vi "test Inhibit Bus A - Single RT.vi"(8 "error in (no error)":errorcluster, 11 "RT Inhibit Bus A in":refnum<class "RT Inhibit Bus A.lvclass">) -> (0 "error out":errorcluster, 3 "RT Inhibit Bus A out":refnum<class "RT Inhibit Bus A.lvclass">)   [LabVIEW 2016, in "RT Inhibit Bus A.lvclass"]
uses:
  RT Inhibit Bus A.lvclass
  1553 Board/1553 Board.lvclass
  1553 Component/1553 Component.lvclass
  Remote Terminal/Remote Terminal.lvclass
  Remote Terminal/TypeDefs/RT Configuration.ctl
  1553 SubComponent/TypeDefs/Scaling Information.ctl
  1553 SubComponent/1553 SubComponent.lvclass
  1553 SubComponent/TypeDefs/Parameter Table Data.ctl
  Remote Terminal/TypeDefs/Command Type.ctl
  Remote Terminal/TypeDefs/Command Configuration.ctl
  PPLs/FPGA Interface.lvlibp/FPGA Interface/FPGA Interface.lvclass
  D:/SVN/Products/BCI-1553/Software/Development/2016/RealTime/1553 SubComponent/1553 SubComponent.lvclass
  Utilities/FPGA Interface/FPGA Interface.lvclass
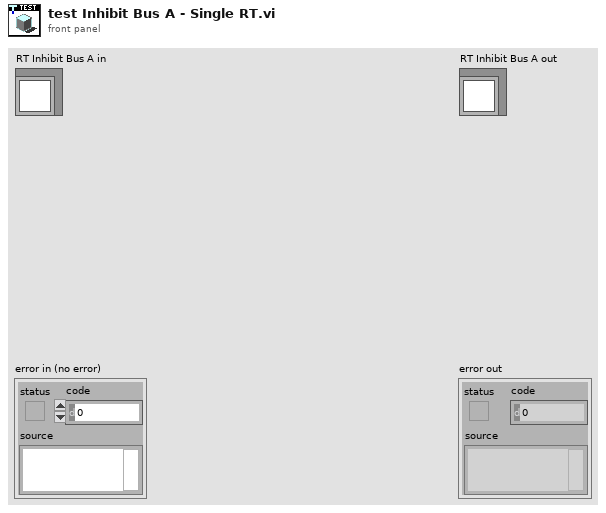
[diagram p1: front panel]
types:
  T1 = typedef "BCI-1553 API.lvlib/Remote Terminal.lvclass/Command Configuration.ctl" = cluster{"Command Type":T2, "Mode Code ID (1-32)":u16, "SubAddress (1-30)":u16, "Word Count (1-32)":u16, "Illegal Command":bool, "Broadcast":bool, "Data":u16[], "Data Fields":T3[]}
  T2 = typedef "BCI-1553 API.lvlib/Remote Terminal.lvclass/Command Type.ctl" = enum16{"Transmit", "Receive", "Mode Code Tx", "Mode Code Rx"}
  T3 = typedef "BCI-1553 API.lvlib/1553 SubComponent.lvclass/Parameter Table Data.ctl" = cluster{"Parameter Name":string, "Base Word":u16, "Address":u16, "Value":u64, "Mask":u16[], "Scaling Info":T4}
  T4 = typedef "BCI-1553 API.lvlib/1553 SubComponent.lvclass/Scaling Information.ctl" = cluster{"Bit Offset":i32, "Bit Count":i32, "LSB Resolution":dbl, "2's Complement":bool, "Big Endian":bool, "Sign Bit":bool}
  T5 = typedef "BCI-1553 API.lvlib/Remote Terminal.lvclass/RT Configuration.ctl" = cluster{"RT-RT TimeOut (us)":u8, "Inhibit Bus A":bool, "Inhibit Bus B":bool, "Broadcast CMD Invalid":bool, "UnDef MCs Invalid":bool, "Notice 2 Data Storage":bool, "SMCP":bool, "Temp RX Buffer":bool, "Alt BIT Enable":bool, "Auto Bus Shutdown":bool, "MC 17 Sync":u8, "MC 16 SR Reset":bool, "MC 8 Reset":bool}
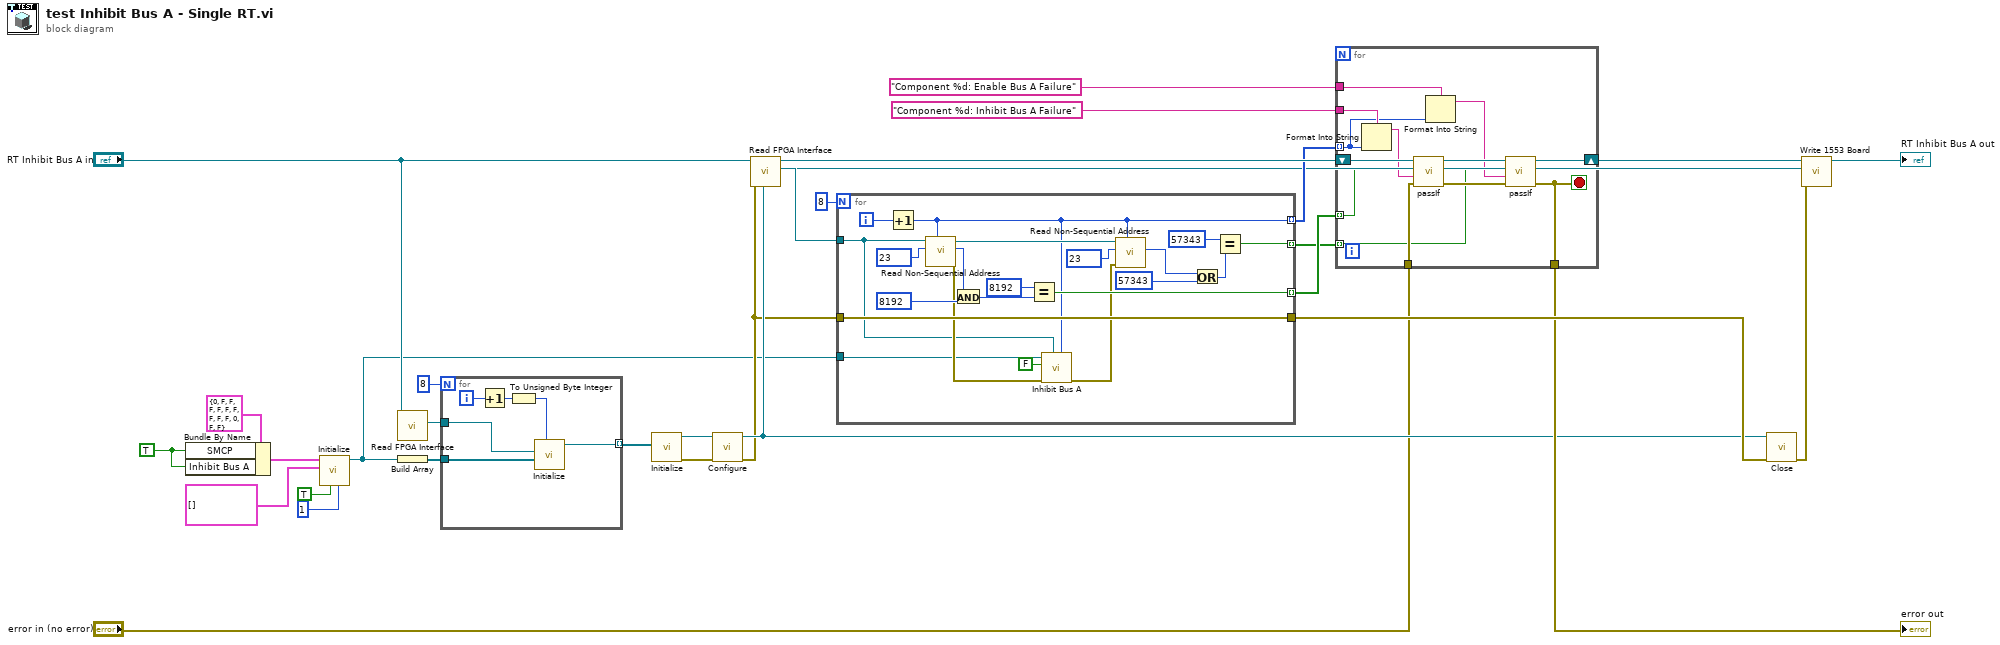
[diagram p0: block diagram]
diagram:
  w21 = TRUE ("SMCP")
  n1 = Bundle By Name(cluster=T5 {"RT-RT TimeOut (us)"=0, "Inhibit Bus A"=FALSE, "Inhibit Bus B"=FALSE, "Broadcast CMD Invalid"=FALSE, "UnDef MCs Invalid"=FALSE, "Notice 2 Data Storage"=FALSE, "SMCP"=FALSE, "Temp RX Buffer"=FALSE, "Alt BIT Enable"=FALSE, "Auto Bus Shutdown"=FALSE, "MC 17 Sync"=0, "MC 16 SR Reset"=FALSE, "MC 8 Reset"=FALSE} ("RT Configuration"), "SMCP"=w21, "Inhibit Bus A"=w21) -> (w28:T5)
  n2 = call "Initialize.vi"("RT Address (0-30)"=u8 1, "RT 1?"=TRUE, "Commands"=T1[] [], "RT Configuration"=w28) -> ("Remote Terminal out"=w3:refnum<class "Remote Terminal.lvclass">)  [unwired: 6 in, 1 out]
  n3 = call-dynamic "Read FPGA Interface.vi"("1553 Test in"="RT Inhibit Bus A in") -> ("FPGA Interface"=w26:refnum<class "FPGA Interface.lvclass">)  [unwired: 8 in, 2 out]
  n4 = Build Array(w3) -> (w27:refnum<class "Remote Terminal.lvclass">[])
  n5 = for {
    N: 8 -> [_]
    tunnel: [w34] -> w30 mode=indexing
    tunnel: w27 -> [w33]
    tunnel: w26 -> [w32]
    i -> [w36]
    n6 = Increment(x=w36) -> (x+1=w31:i32)
    n7 = To Unsigned Byte Integer(number=w31) -> (unsigned 8bit integer=w35:u8)
    n8 = call "Initialize.vi"("Component ID (1-8)"=w35, "SubComponents"=w33, "FPGA Interface"=w32) -> ("1553 Component out"=w34:refnum<class "1553 Component.lvclass">)  [unwired: 7 in, 1 out]
  }
  n9 = call "Initialize.vi"("Components"=w30) -> ("error out"=w6:errorcluster, "1553 Board out"=w8:refnum<class "1553 Board.lvclass">)  [unwired: 9 in]
  n10 = call-dynamic "Configure.vi"("error in (no error)"=w6, "1553 Board in"=w8) -> ("error out"=w5:errorcluster, "1553 Board out"=w7:refnum<class "1553 Board.lvclass">)  [unwired: 8 in]
  n11 = call-dynamic "Read FPGA Interface.vi"("error in (no error)"=w5, "1553 Test in"="RT Inhibit Bus A in") -> ("FPGA Interface"=w16:refnum<class "FPGA Interface.lvclass">, "1553 Test out"=w15:refnum<class "RT Inhibit Bus A.lvclass">)  [unwired: 7 in, 1 out]
  n12 = for {
    N: 8 -> [_]
    tunnel: w5 -> [w50]
    tunnel: [w50] -> w17
    tunnel: w16 -> [w45]
    tunnel: [w49] -> w13 mode=indexing
    tunnel: [w44] -> w10 mode=indexing
    tunnel: w3 -> [w47]
    tunnel: [w41] -> w1 mode=indexing
    i -> [w51]
    n13 = Increment(x=w51) -> (x+1=w44:i32)
    n14 = call-dynamic "Read Non-Sequential Address.vi"("Target IC (1-8)"=w44, "Address"=u16 23, "FPGA Interface in"=w45) -> ("error out"=w48:errorcluster, "Data"=w52:u16)  [unwired: 7 in]
    n15 = And(x=w52, y=u16 8192) -> (x .and. y?=w53:u16)
    n16 = Equal?(x=u16 8192, y=w53) -> (x = y?=w49:bool)
    n17 = call-dynamic "Inhibit Bus A.vi"("Component ID"=w44, "FPGA Interface"=w45, "error in (no error)"=w48, "Inhibit Bus A?"=FALSE, "Remote Terminal in"=w47) -> ("error out"=w42:errorcluster)  [unwired: 5 in, 1 out]
    n18 = call-dynamic "Read Non-Sequential Address.vi"("Target IC (1-8)"=w44, "error in (no error)"=w42, "Address"=u16 23, "FPGA Interface in"=w45) -> ("Data"=w38:u16)  [unwired: 6 in, 1 out]
    n19 = Or(x=w38, y=u16 57343) -> (x .or. y?=w37:u16)
    n20 = Equal?(x=u16 57343, y=w37) -> (x = y?=w41:bool)
  }
  n21 = for {
    shift-right: [w61] -> w14
    shift-left: w15 -> [w69]
    tunnel: w13 -> [w68] mode=indexing
    tunnel: [w59] -> w12
    tunnel: "Component %d: Inhibit Bus A Failure" ("custom report message (\"\")") -> [w67]
    tunnel: w10 -> [w63] mode=indexing
    tunnel: "error in (no error)" -> [w65]
    tunnel: "Component %d: Enable Bus A Failure" ("custom report message (\"\")") -> [w64]
    tunnel: w1 -> [w57] mode=indexing
    stop <- w59 stop-if-true
    n22 = Format Into String(format string=w67, w63) -> (resulting string=w66:string)  [unwired: 2 in, 1 out]
    n23 = call-dynamic "passIf.vi"("error in (no error)"=w65, "message (\"\")"=w66, "pass"=w68, "TestCase in"=w69) -> ("error out"=w60:errorcluster, "TestCase out"=w62:refnum<class "RT Inhibit Bus A.lvclass">)  [unwired: 6 in]
    n24 = Format Into String(format string=w64, w63) -> (resulting string=w58:string)  [unwired: 2 in, 1 out]
    n25 = call-dynamic "passIf.vi"("error in (no error)"=w60, "message (\"\")"=w58, "pass"=w57, "TestCase in"=w62) -> ("error out"=w59:errorcluster, "TestCase out"=w61:refnum<class "RT Inhibit Bus A.lvclass">)  [unwired: 6 in]
  }
  "error out" <- w12
  n26 = call-dynamic "Close.vi"("error in (no error)"=w17, "1553 Board in"=w7) -> ("error out"=w18:errorcluster)  [unwired: 9 in]
  n27 = call-dynamic "Write 1553 Board.vi"("error in (no error)"=w18, "1553 Board"=w7, "1553 Test in"=w14) -> ("1553 Test out"=→"RT Inhibit Bus A out":refnum<class "RT Inhibit Bus A.lvclass">)  [unwired: 7 in, 1 out]
